vi "DAQ Write.vi"(8 "error in (no error)":errorcluster, 10 "Outputs":dbl[](array[numeric]), 11 "DAQ Tasks":T1) -> (0 "error out":errorcluster, 3 "dup DAQ Tasks":T1)   [LabVIEW 2017]
uses:
  controls/DAQ Tasks.ctl
  <vilib>/DAQmx/write.llb/DAQmx Write.vi
  <vilib>/DAQmx/miscellaneous.llb/DAQmx Fill In Error Info.vi
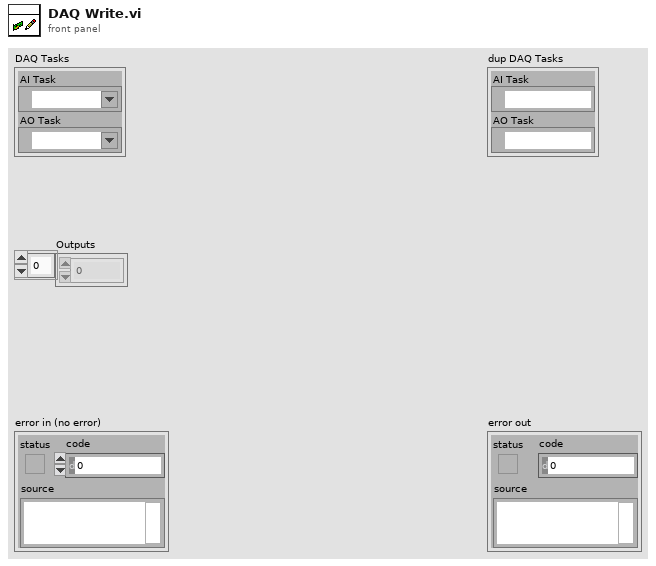
[diagram p1: front panel]
types:
  T1 = typedef "DAQ Tasks.ctl" = cluster{"AI Task":refnum<k21>, "AO Task":refnum<k21>}
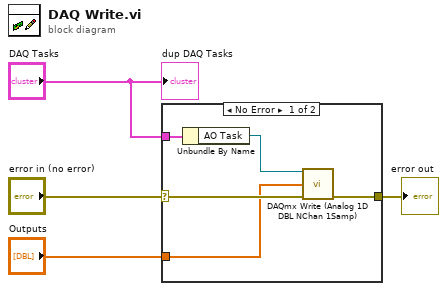
[diagram p0: block diagram]
diagram:
  n1 = case shown="No Error" "error in (no error)" {
    selector: "error in (no error)" -> [w6 w10]
    tunnel: [w9 w10] -> w4
    tunnel: "DAQ Tasks" -> [w7 _]
    tunnel: "Outputs" -> [w5 _]
    frame No Error {
      n2 = Unbundle By Name(w7) -> ("AO Task"=w8:refnum<k21>)
      n3 = call-poly <vilib>:"DAQmx Write (Analog 1D DBL NChan 1Samp).vi"("task/channels in"=w8, "data"=w5, "error in"=w6) -> ("error out"=w9:errorcluster)  [unwired: 10 in, 2 out]
    }
    frame Error {
    }
  }
  "error out" <- w4
  "dup DAQ Tasks" <- "DAQ Tasks"
